vi "RefreshCacheMap.vi"(8 "error in (no error)":errorcluster, 11 "UserEventTimer in":refnum<class "TimerEngine.lvclass">) -> (0 "error out":errorcluster, 3 "UserEventTimer out":refnum<class "TimerEngine.lvclass">)   [LabVIEW 2017, in "TimerEngine.lvlib" / "TimerEngine.lvclass"]
uses:
  TimerEngine.lvclass
  TimerEngine.lvclass/TimerEngine.ctl
  _TimerClass/Timer.lvclass/Timer.ctl
  _TimerClass/Timer.lvclass
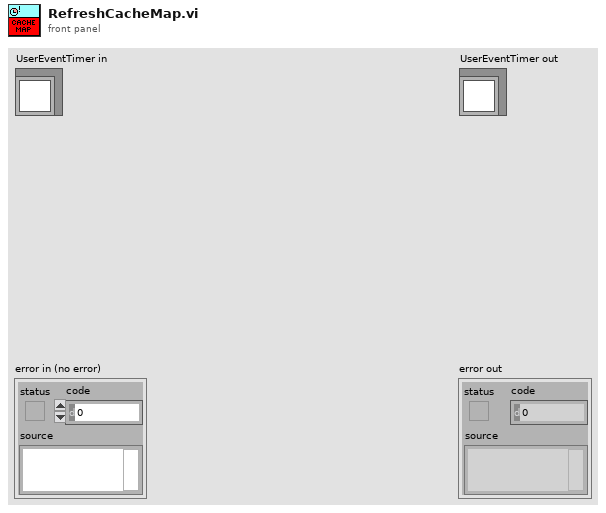
[diagram p1: front panel]
types:
  T1 = typedef "TimerEngine.lvlib/TimerEngine.lvclass/Timer-UserEvent.ctl" = refnum<user-event>
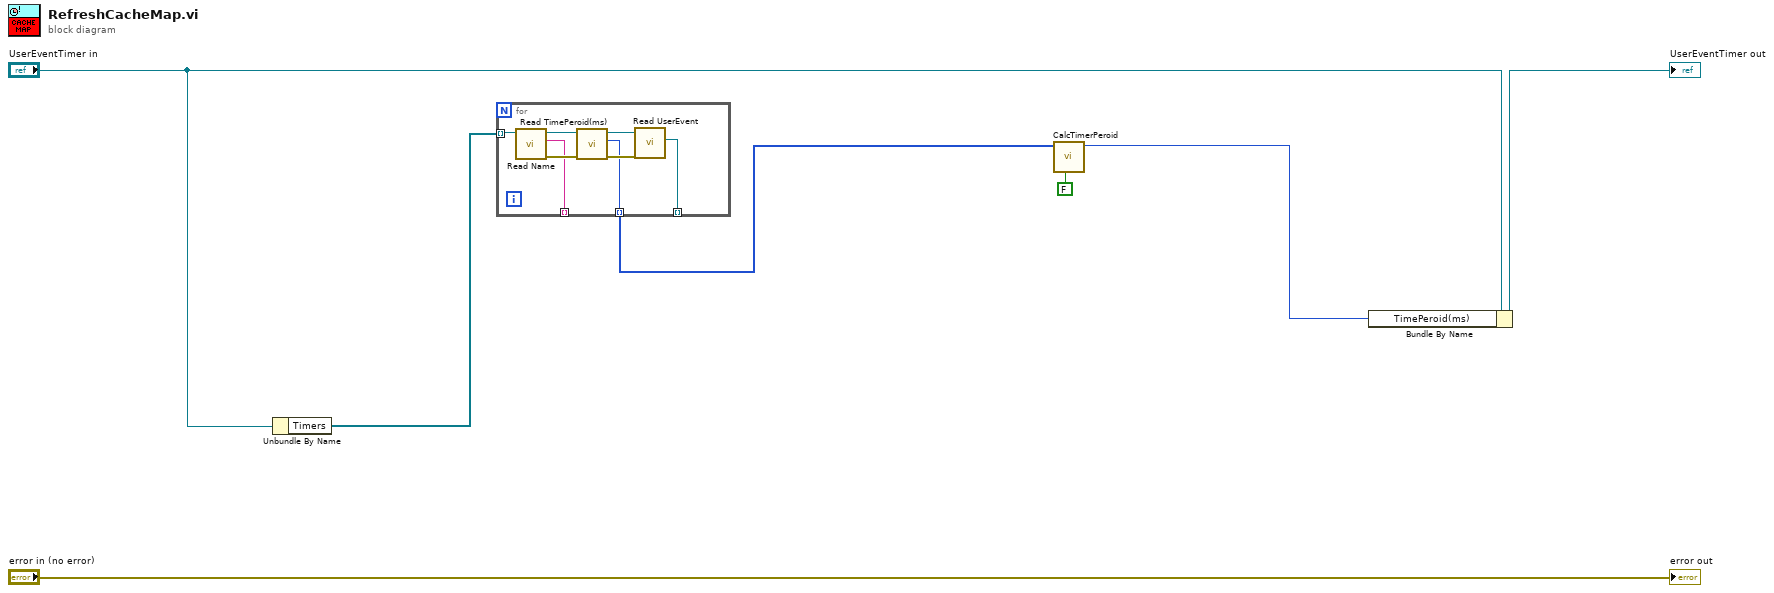
[diagram p0: block diagram]
diagram:
  n1 = Unbundle By Name("UserEventTimer in") -> ("Timers"=w2:refnum<class "Timer.lvclass">[])
  n2 = for {
    tunnel: w2 -> [w15] mode=indexing
    tunnel: [w10] -> _ mode=indexing
    tunnel: [w9] -> w1 mode=indexing
    tunnel: [w8] -> _ mode=indexing
    n3 = call "Read Name.vi"("Timer in"=w15) -> ("error out"=w11:errorcluster, "Name"=w10:string, "Timer out"=w14:refnum<class "Timer.lvclass">)  [unwired: 8 in]
    n4 = call "Read TimePeroid(ms).vi"("error in (no error)"=w11, "Timer in"=w14) -> ("error out"=w13:errorcluster, "TimePeroid(ms)"=w9:i64, "Timer out"=w12:refnum<class "Timer.lvclass">)  [unwired: 7 in]
    n5 = call "Read UserEvent.vi"("error in (no error)"=w13, "Timer in"=w12) -> ("UserEvent"=w8:T1)  [unwired: 7 in, 2 out]
  }
  n6 = call "CalcTimerPeroid.vi"("Exclude Inputs?"=FALSE, "TimePeroid"=w1) -> ("Proper TimePeroid"=w3:i32)  [unwired: 9 in]
  n7 = Bundle By Name(cluster="UserEventTimer in", "TimePeroid(ms)"=w3) -> (→"UserEventTimer out":refnum<class "TimerEngine.lvclass">)
  "error out" <- "error in (no error)"
